vi "Notify Observers (State).vi"(8 "error in (no error)":errorcluster, 10 "State Message":refnum<class "MSG.lvclass">, 11 "ObserverRegistry in":refnum<class "ObserverRegistry.lvclass">) -> (0 "error out":errorcluster, 3 "ObserverRegistry out":refnum<class "ObserverRegistry.lvclass">)   [LabVIEW 2011, in "Messenging.lvlib" / "ObserverRegistry.lvclass"]
uses:
  ObserverRegistry.lvclass
  Interprocess Messenger/TextVarientMessage/MSG.lvclass
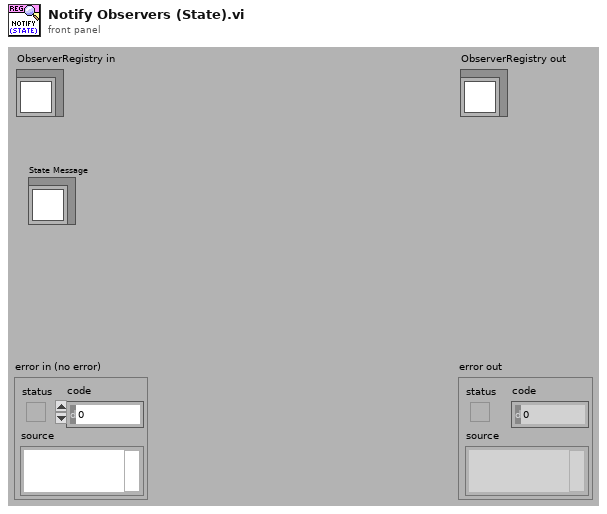
[diagram p1: front panel]
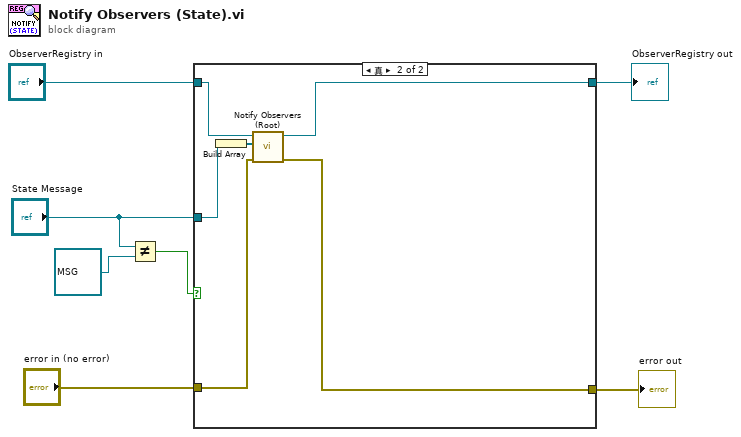
[diagram p0: block diagram]
diagram:
  n1 = Not Equal?(x="State Message", y=refnum<class "MSG.lvclass"> refnum ("Message")) -> (x != y?=w1:bool)
  n2 = case shown="真" w1 {
    tunnel: "ObserverRegistry in" -> [w9 w13]
    tunnel: [w9 w11] -> w6
    tunnel: "error in (no error)" -> [w8 w12]
    tunnel: [w8 w10] -> w4
    tunnel: "State Message" -> [_ w15]
    frame False {
      # "Null Message"
    }
    frame True {
      n3 = Build Array(w15) -> (w14:refnum<class "MSG.lvclass">[])
      n4 = call "Notify Observers (Root).vi"("error in (no error)"=w12, "Array of State Messages"=w14, "ObserverRegistry in"=w13) -> ("error out"=w10:errorcluster, "ObserverRegistry out"=w11:refnum<class "ObserverRegistry.lvclass">)  [unwired: 1 in, 6 out]
    }
  }
  "error out" <- w4
  "ObserverRegistry out" <- w6
